vi "Add_Run_info.vi"() -> (5 "Plug in titles":string[](array[string]), 7 "Plug in values":string[](array[string]))   [LabVIEW 2010]
uses:
  Globals/Meas_global.vi
panel:
  in  "OK":bool
  in  "Plug in values In":string[](array[string])=["2915", "0"]
  in  "Plug in titles In":string[](array[string])=["Floating:Floor:Center X (mm)", "Cantilever:Deflection:(mm)"]
  # "Please enter any run information in the box below"
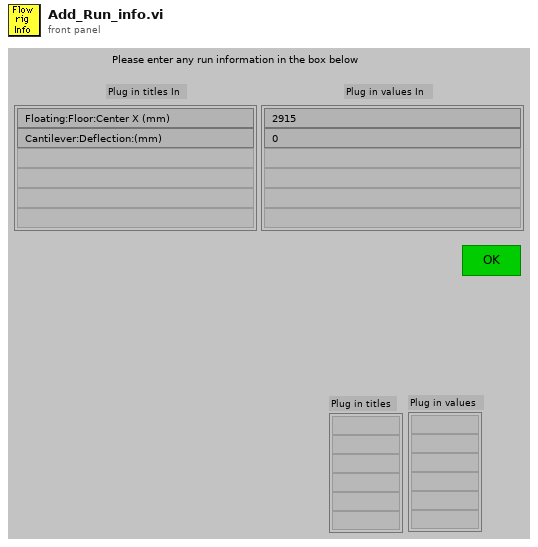
[diagram p1: front panel]
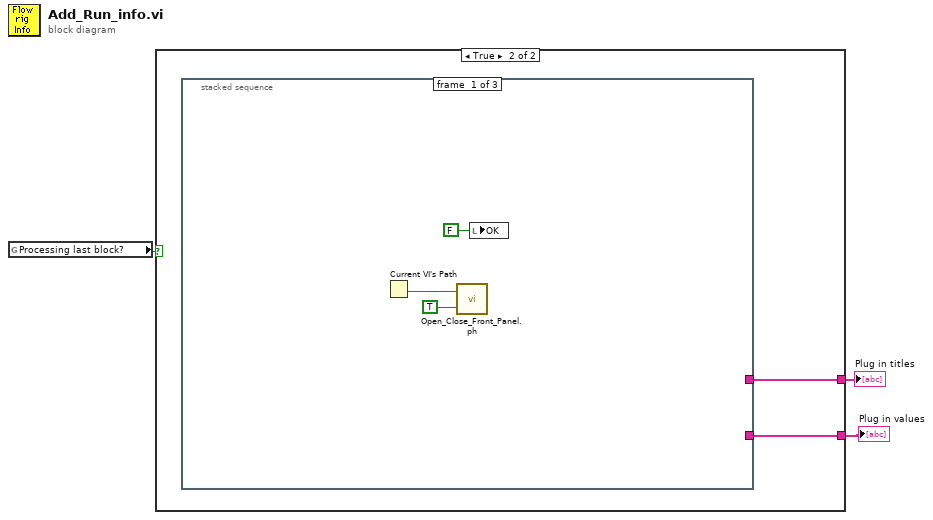
[diagram p0: block diagram]
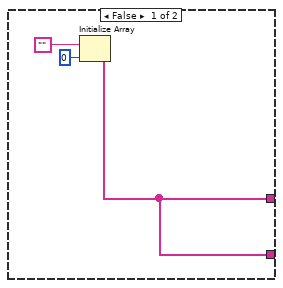
[diagram p2: hidden frame]
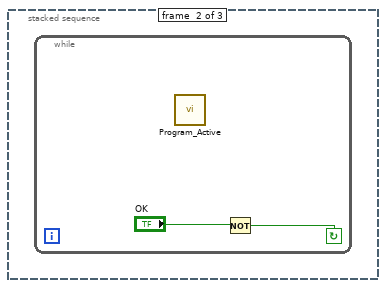
[diagram p3: hidden frame]
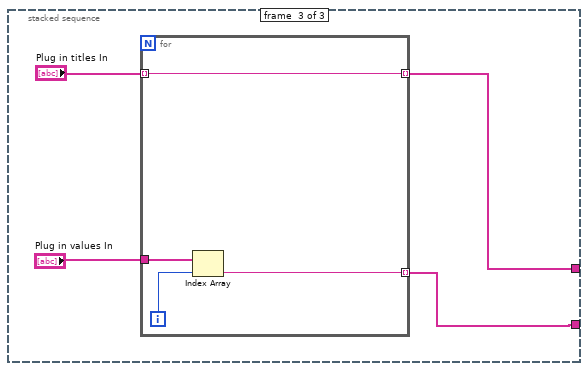
[diagram p4: hidden frame]
diagram:
  n1 = global read "Meas_global.vi" "Processing last block?"() -> (w3:bool)
  n2 = case shown="True" w3 {
    tunnel: [w4 w7] -> w2
    tunnel: [w4 w8] -> w1
    frame False {
      n3 = Initialize Array("", 0) -> (w4:string[])
    }
    frame True {
      n4 = stacked-sequence {
        tunnel: [_ _ w14] -> w8
        tunnel: [_ _ w17] -> w7
        frame #0 {
          n5 = Current VI's Path() -> (path=w10:path)
          n6 = call "Open_Close_Front_Panel.ph.vi"("Front Panel Window:Open"=TRUE, "VI path"=w10) -> ()  [unwired: 2 out]
          n7 = local write "OK"(FALSE ("OK")) -> ()
        }
        frame #1 {
          n8 = while {
            stop <- w12 continue-if-true
            n9 = call "Program_Active.vi"() -> ()  [unwired: 1 in]
            n10 = Not(x="OK") -> (.not. x?=w12:bool)
          }
        }
        frame #2 {
          n11 = for {
            tunnel: [w21] -> w17 mode=indexing
            tunnel: "Plug in titles In" -> [w21] mode=indexing
            tunnel: "Plug in values In" -> [w19]
            tunnel: [w18] -> w14 mode=indexing
            i -> [w20]
            n12 = Index Array(array=w19, index=w20) -> (element=w18:string)
          }
        }
      }
    }
  }
  "Plug in titles" <- w2
  "Plug in values" <- w1
